vi "File & Folder IG.vi"(8 "error in (no error)":errorcluster) -> (0 "error out":errorcluster, 3 "Cluster 2":T1)   [LabVIEW 2022 SP3]
uses:
  Controls/file folder ctll.ctl
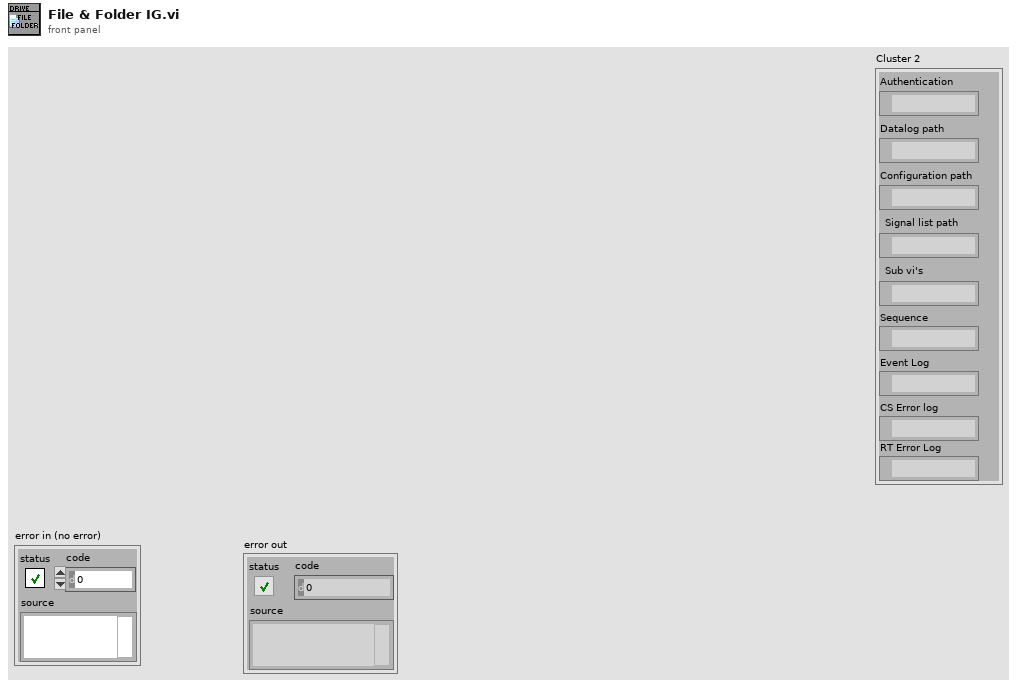
[diagram p1: front panel]
types:
  T1 = typedef "file folder ctll.ctl" = cluster{"Datalog path":path, "Configuration path":path, "Signal list path":path, "Sub vi's":path, "Authentication":path, "Sequence":path, "Event Log":path, "CS Error log":path, "RT Error Log":path}
  T2 = enum32{"invalid app kind", "Development System", "Run Time System", "Student Edition", "Embedded LabVIEW", "Evaluation", "Custom"}
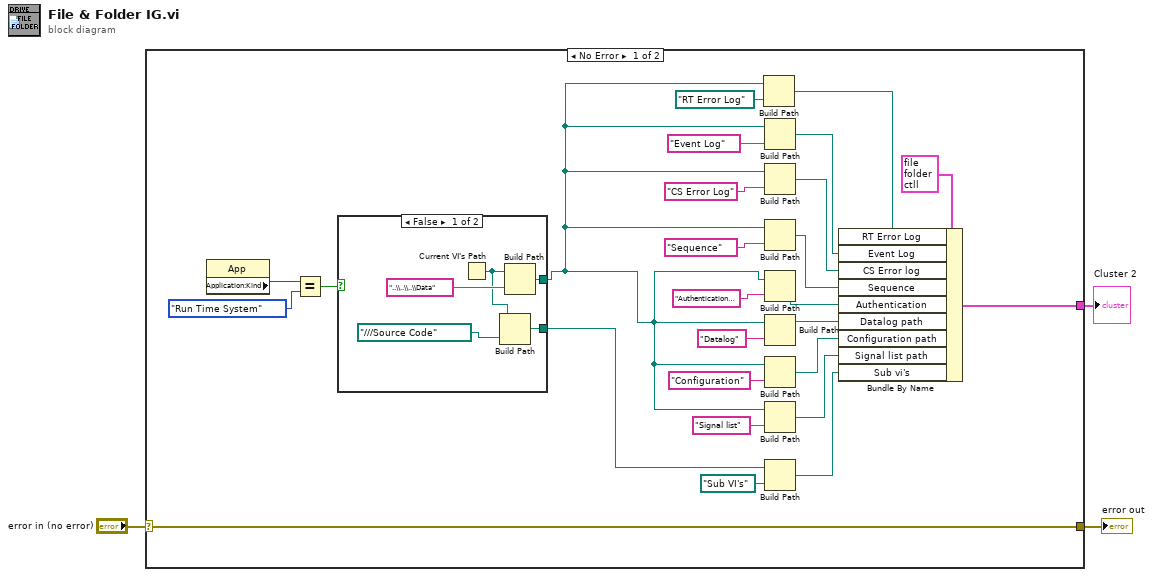
[diagram p0: block diagram]
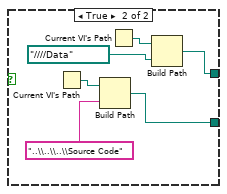
[diagram p2: hidden frame]
diagram:
  n1 = case shown="No Error" "error in (no error)" {
    selector: "error in (no error)" -> [w26 _]
    tunnel: [w26 _] -> w2
    tunnel: [w25 _] -> w1
    frame No Error {
      n2 = property class="App"() -> ("Application:Kind"=w8:T2)  [unwired: 2 in, 2 out]
      n3 = Equal?(x=w8, y=T2."Run Time System") -> (x = y?=w6:bool)
      n4 = case shown="False" w6 {
        tunnel: [w33 w37] -> w5
        tunnel: [w30 w35] -> w4
        frame False {
          n5 = Current VI's Path() -> (path=w32:path)
          n6 = Build Path(base path=w32, name or relative path=path "../../../Source Code" ("appended path")) -> (appended path=w30:path)
          n7 = Build Path(base path=w32, name or relative path="..\\..\\..\\Data") -> (appended path=w33:path)
        }
        frame True {
          n8 = Current VI's Path() -> (path=w40:path)
          n9 = Build Path(base path=w40, name or relative path="..\\..\\..\\Source Code") -> (appended path=w35:path)
          n10 = Current VI's Path() -> (path=w38:path)
          n11 = Build Path(base path=w38, name or relative path=path "../../../../Data" ("appended path")) -> (appended path=w37:path)
        }
      }
      n12 = Build Path(base path=w5, name or relative path=path "RT Error Log") -> (appended path=w9:path)
      n13 = Build Path(base path=w5, name or relative path="Event Log") -> (appended path=w12:path)
      n14 = Build Path(base path=w5, name or relative path="CS Error Log") -> (appended path=w11:path)
      n15 = Build Path(base path=w5, name or relative path="Sequence") -> (appended path=w15:path)
      n16 = Build Path(base path=w5, name or relative path="Authentication Details") -> (appended path=w17:path)
      n17 = Build Path(base path=w5, name or relative path="Datalog") -> (appended path=w27:path)
      n18 = Build Path(base path=w5, name or relative path="Configuration") -> (appended path=w22:path)
      n19 = Build Path(base path=w5, name or relative path="Signal list") -> (appended path=w21:path)
      n20 = Build Path(base path=w4, name or relative path=path "Sub VI's") -> (appended path=w19:path)
      n21 = Bundle By Name(cluster=T1 {"Datalog path"=path "", "Configuration path"=path "", "Signal list path"=path "", "Sub vi's"=path "", "Authentication"=path "", "Sequence"=path "", "Event Log"=path "", "CS Error log"=path "", "RT Error Log"=path ""} ("Cluster 2"), "RT Error Log"=w9, "Event Log"=w12, "CS Error log"=w11, "Sequence"=w15, "Authentication"=w17, "Datalog path"=w27, "Configuration path"=w22, "Signal list path"=w21, "Sub vi's"=w19) -> (w25:T1)
    }
    frame Error {
    }
  }
  "error out" <- w2
  "Cluster 2" <- w1
